vi "FindNearestPointOnCuboid.vi"(10 "3D Cuboid":T2, 11 "3D Point":T1) -> (3 "Nearest Point":T1)   [LabVIEW 2020]
uses:
  3Dpoint.ctl
  3DCuboid.ctl
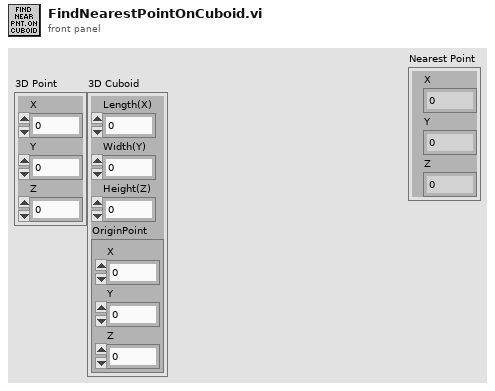
[diagram p1: front panel]
types:
  T1 = typedef "3Dpoint.ctl" = cluster{"X":dbl, "Y":dbl, "Z":dbl}
  T2 = typedef "3DCuboid.ctl" = cluster{"Length(X)":dbl, "Width(Y)":dbl, "Height(Z)":dbl, "OriginPoint":T1}
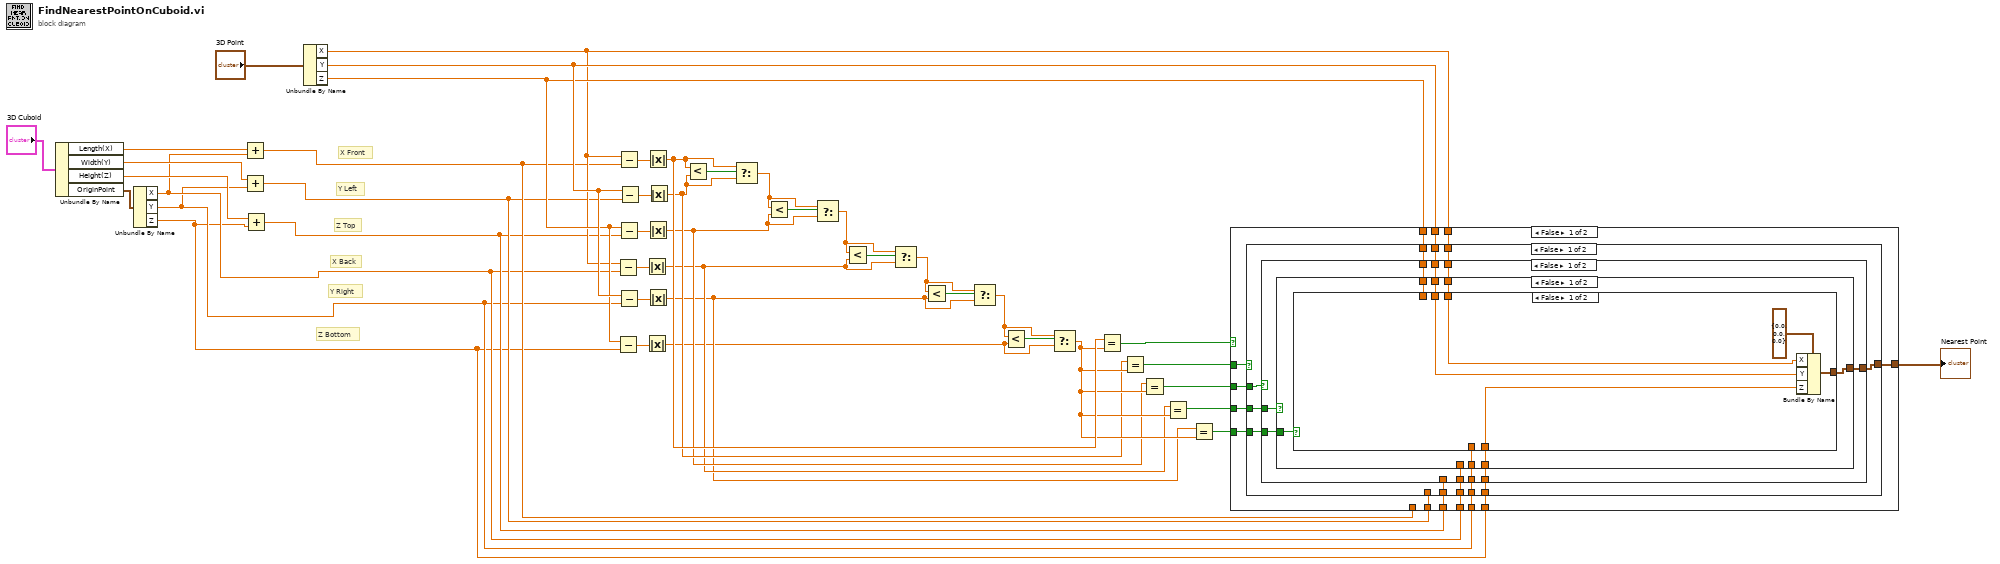
[diagram p0: block diagram]
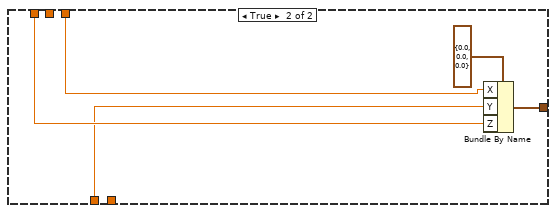
[diagram p2: hidden frame]
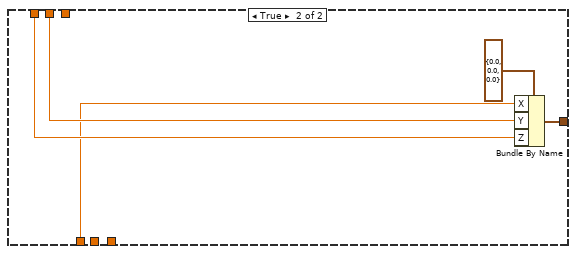
[diagram p3: hidden frame]
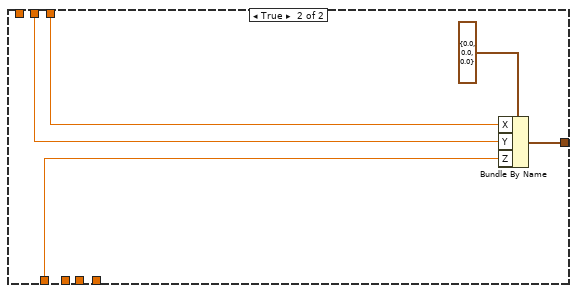
[diagram p4: hidden frame]
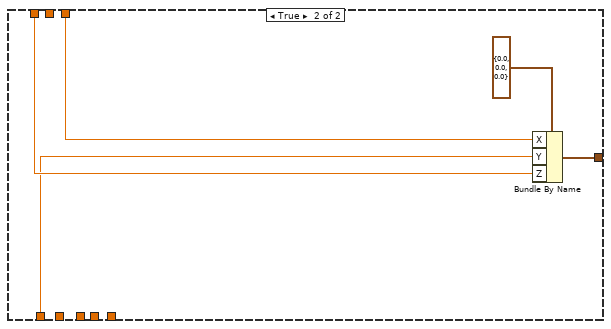
[diagram p5: hidden frame]
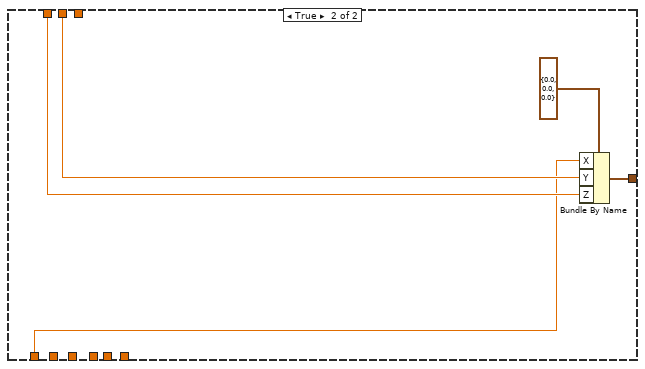
[diagram p6: hidden frame]
diagram:
  # "Y Left"
  # "X Front"
  # "Z Top"
  # "Z Bottom"
  # "Y Right"
  # "X Back"
  n1 = Unbundle By Name("3D Cuboid") -> ("Length(X)"=w39:dbl, "Width(Y)"=w40:dbl, "Height(Z)"=w38:dbl, "OriginPoint"=w41:T1)
  n2 = Unbundle By Name(w41) -> ("X"=w7:dbl, "Y"=w6:dbl, "Z"=w5:dbl)
  n3 = Add(x=w39, y=w7) -> (x+y=w10:dbl)
  n4 = Add(x=w40, y=w6) -> (x+y=w9:dbl)
  n5 = Add(x=w38, y=w5) -> (x+y=w8:dbl)
  n6 = Unbundle By Name("3D Point") -> ("X"=w11:dbl, "Y"=w13:dbl, "Z"=w12:dbl)
  n7 = Subtract(x=w11, y=w7) -> (x-y=w31:dbl)
  n8 = Subtract(x=w12, y=w5) -> (x-y=w29:dbl)
  n9 = Subtract(x=w11, y=w10) -> (x-y=w36:dbl)
  n10 = Subtract(x=w12, y=w8) -> (x-y=w32:dbl)
  n11 = Subtract(x=w13, y=w6) -> (x-y=w30:dbl)
  n12 = Subtract(x=w13, y=w9) -> (x-y=w35:dbl)
  n13 = Absolute Value(x=w31) -> (abs(x)=w18:dbl)
  n14 = Absolute Value(x=w29) -> (abs(x)=w16:dbl)
  n15 = Absolute Value(x=w36) -> (abs(x)=w22:dbl)
  n16 = Absolute Value(x=w32) -> (abs(x)=w19:dbl)
  n17 = Absolute Value(x=w30) -> (abs(x)=w17:dbl)
  n18 = Absolute Value(x=w35) -> (abs(x)=w20:dbl)
  n19 = Less?(x=w22, y=w20) -> (x < y?=w37:bool)
  n20 = Select(t=w22, s=w37, f=w20) -> (s? t:f=w33:dbl)
  n21 = Less?(x=w33, y=w19) -> (x < y?=w34:bool)
  n22 = Select(t=w33, s=w34, f=w19) -> (s? t:f=w27:dbl)
  n23 = Less?(x=w27, y=w18) -> (x < y?=w28:bool)
  n24 = Select(t=w27, s=w28, f=w18) -> (s? t:f=w23:dbl)
  n25 = Less?(x=w23, y=w17) -> (x < y?=w26:bool)
  n26 = Select(t=w23, s=w26, f=w17) -> (s? t:f=w24:dbl)
  n27 = Less?(x=w24, y=w16) -> (x < y?=w25:bool)
  n28 = Select(t=w24, s=w25, f=w16) -> (s? t:f=w21:dbl)
  n29 = Equal?(x=w22, y=w21) -> (x = y?=w15:bool)
  n30 = Equal?(x=w20, y=w21) -> (x = y?=w4:bool)
  n31 = Equal?(x=w19, y=w21) -> (x = y?=w3:bool)
  n32 = Equal?(x=w18, y=w21) -> (x = y?=w2:bool)
  n33 = Equal?(x=w17, y=w21) -> (x = y?=w1:bool)
  n34 = case shown="False" w15 {
    tunnel: [w52 w112] -> w14
    tunnel: w13 -> [w48 w111]
    tunnel: w12 -> [w50 w110]
    tunnel: w11 -> [w51 _]
    tunnel: w10 -> [_ w109]
    tunnel: w9 -> [w49 _]
    tunnel: w8 -> [w47 _]
    tunnel: w7 -> [w46 _]
    tunnel: w6 -> [w45 _]
    tunnel: w5 -> [w44 _]
    tunnel: w4 -> [w56 _]
    tunnel: w3 -> [w55 _]
    tunnel: w2 -> [w54 _]
    tunnel: w1 -> [w53 _]
    frame False {
      n35 = case shown="False" w56 {
        tunnel: w55 -> [w67 _]
        tunnel: w54 -> [w66 _]
        tunnel: w53 -> [w65 _]
        tunnel: [w64 w107] -> w52
        tunnel: w51 -> [w63 w106]
        tunnel: w50 -> [w60 w105]
        tunnel: w49 -> [_ w104]
        tunnel: w48 -> [w62 _]
        tunnel: w47 -> [w61 _]
        tunnel: w46 -> [w59 _]
        tunnel: w45 -> [w58 _]
        tunnel: w44 -> [w57 _]
        frame False {
          n36 = case shown="False" w67 {
            tunnel: w66 -> [w76 _]
            tunnel: w65 -> [w75 _]
            tunnel: [w74 w102] -> w64
            tunnel: w63 -> [w70 w101]
            tunnel: w62 -> [w73 w100]
            tunnel: w61 -> [_ w99]
            tunnel: w60 -> [w72 _]
            tunnel: w59 -> [w71 _]
            tunnel: w58 -> [w69 _]
            tunnel: w57 -> [w68 _]
            frame False {
              n37 = case shown="False" w76 {
                tunnel: w75 -> [w83 _]
                tunnel: [w82 w97] -> w74
                tunnel: w73 -> [w78 w96]
                tunnel: w72 -> [w80 w95]
                tunnel: w71 -> [_ w94]
                tunnel: w70 -> [w81 _]
                tunnel: w69 -> [w79 _]
                tunnel: w68 -> [w77 _]
                frame False {
                  n38 = case shown="False" w83 {
                    tunnel: [w87 w92] -> w82
                    tunnel: w81 -> [w86 w91]
                    tunnel: w80 -> [_ w90]
                    tunnel: w79 -> [_ w89]
                    tunnel: w78 -> [w85 _]
                    tunnel: w77 -> [w84 _]
                    frame False {
                      n39 = Bundle By Name(cluster=T1 {"X"=0.0, "Y"=0.0, "Z"=0.0} ("3D Point"), "X"=w86, "Y"=w85, "Z"=w84) -> (w87:T1)
                    }
                    frame True {
                      n40 = Bundle By Name(cluster=T1 {"X"=0.0, "Y"=0.0, "Z"=0.0} ("3D Point"), "X"=w91, "Y"=w89, "Z"=w90) -> (w92:T1)
                    }
                  }
                }
                frame True {
                  n41 = Bundle By Name(cluster=T1 {"X"=0.0, "Y"=0.0, "Z"=0.0} ("3D Point"), "X"=w94, "Y"=w96, "Z"=w95) -> (w97:T1)
                }
              }
            }
            frame True {
              n42 = Bundle By Name(cluster=T1 {"X"=0.0, "Y"=0.0, "Z"=0.0} ("3D Point"), "X"=w101, "Y"=w100, "Z"=w99) -> (w102:T1)
            }
          }
        }
        frame True {
          n43 = Bundle By Name(cluster=T1 {"X"=0.0, "Y"=0.0, "Z"=0.0} ("3D Point"), "X"=w106, "Y"=w104, "Z"=w105) -> (w107:T1)
        }
      }
    }
    frame True {
      n44 = Bundle By Name(cluster=T1 {"X"=0.0, "Y"=0.0, "Z"=0.0} ("3D Point"), "X"=w109, "Y"=w111, "Z"=w110) -> (w112:T1)
    }
  }
  "Nearest Point" <- w14
